vi "mqtt example gui3.vi"() -> ()   [LabVIEW 2017]
uses:
  mqtt-LabVIEW/src/class/mqtt/mqttConfigFunction.ctl
  mqtt-LabVIEW/src/class/mqtt/mqtt.lvclass/mqtt.ctl
  mqtt-LabVIEW/src/class/mqtt/mqttTypedef/mqttSubscribeCluster.ctl
  mqtt-LabVIEW/src/class/mqtt/mqttTypedef/mqttQOSlevel.ctl
  Global mqttExample.vi
  mqtt payload to double.vi
  mqtt payload to boolean.vi
  mqtt-LabVIEW/src/class/mqtt/mqtt.lvclass
panel:
  in  "G_send client time":bool
  in  "send client time":bool
  in  "auto reconnect":bool
  out "MQTT Subscribed":bool
  out "MQTT Connection":bool
  out "RX Topic":string
  out "RX Value":string
  in  "boolean control":bool
  out "boolean indicator":bool
  out "numeric indicator":dbl min=24.6 max=310.0 format="%0.3f"
  in  "send instruction":bool
  in  "numeric control":dbl format="%0.3f"
  out "messageID":u16
  out "quit":bool
  # "MQTT related"
  # "Last received message"
  # "Example program functions"
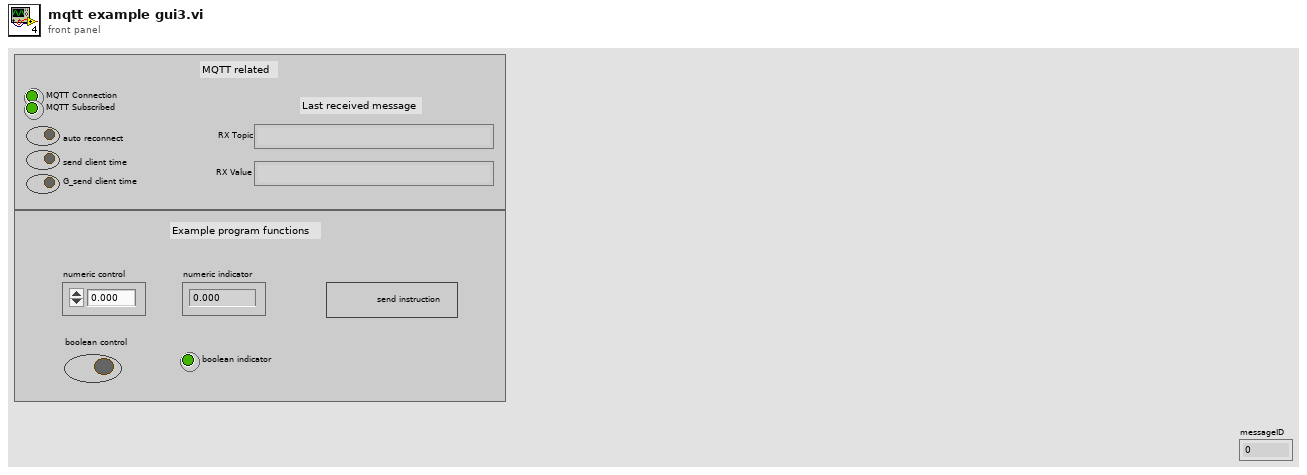
[diagram p1: front panel]
types:
  T1 = enum8{"Enabled", "Disabled", "Disabled and Grayed Out"}
  T2 = typedef "mqtt.lvclass/mqttConfigFunction.ctl" = enum16{"init", "deinit", "set", "get"}
  T3 = typedef "mqttSubscribeCluster.ctl" = cluster{"Topic":string, "QoS":T4}
  T4 = typedef "mqttQOSlevel.ctl" = enum8{"At most once", "At least once", "Exactly once", "Reserved"}
  T5 = typedef "mqttUserInformation.ctl" = cluster{"Will message":string, "Will Topic":string}
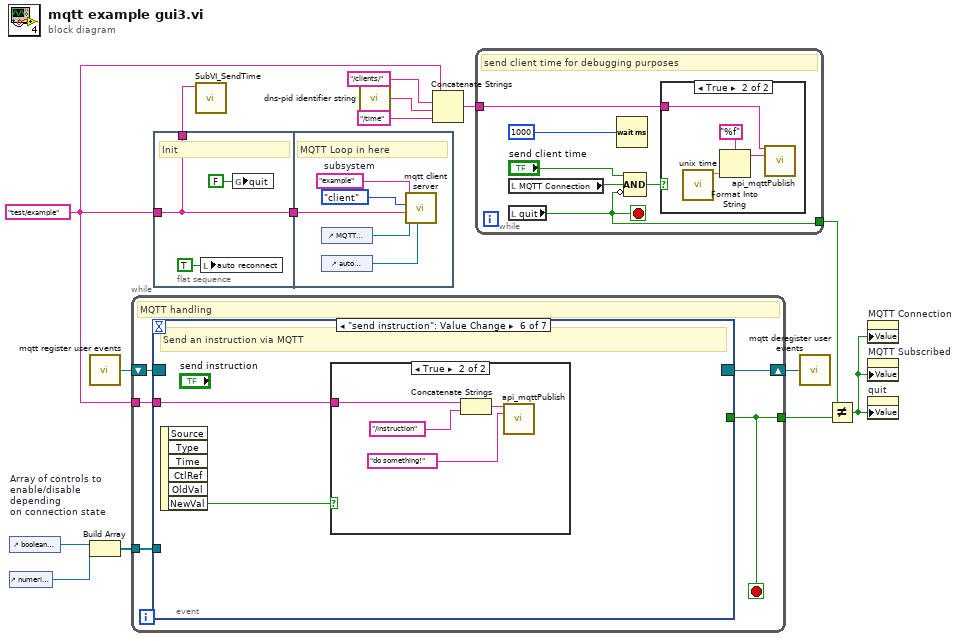
[diagram p0: block diagram]
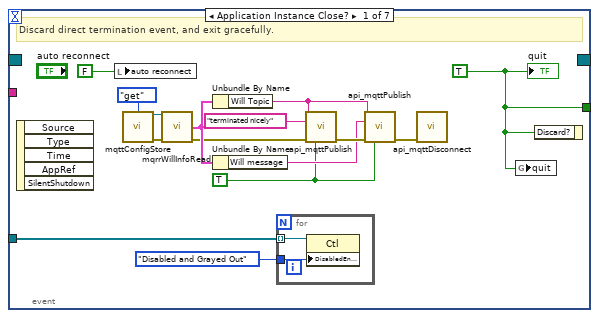
[diagram p3: hidden frame]
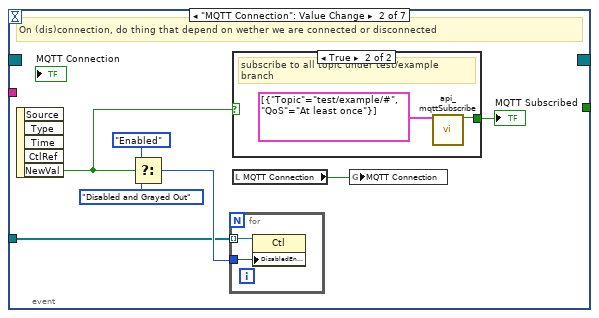
[diagram p4: hidden frame]
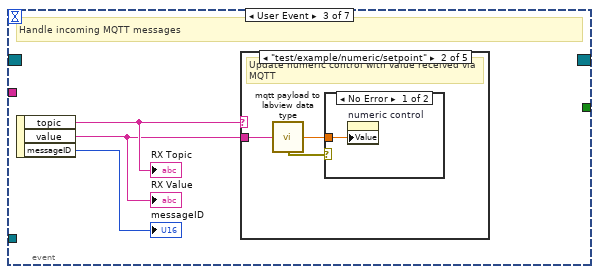
[diagram p6: hidden frame]
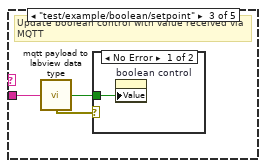
[diagram p9: hidden frame]
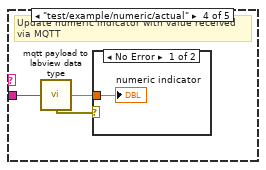
[diagram p11: hidden frame]
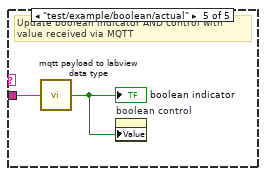
[diagram p13: hidden frame]
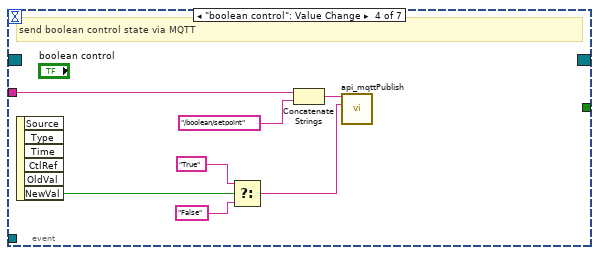
[diagram p14: hidden frame]
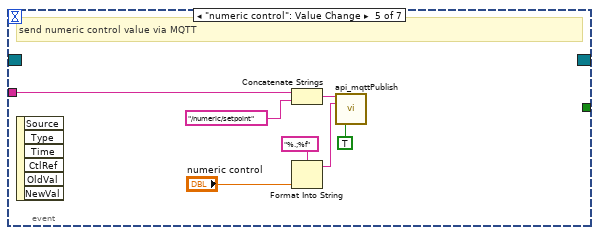
[diagram p15: hidden frame]
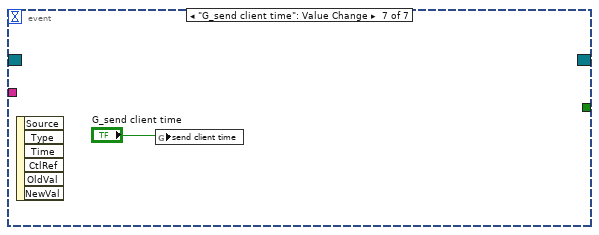
[diagram p17: hidden frame]
diagram:
  w2 = "test/example" ("mqtt prefix")
  n1 = control-ref of="boolean control"() -> (w9:refnum<vi>)
  n2 = control-ref of="numeric control"() -> (w11:refnum<vi>)
  n3 = call "mqtt register user events.vi"() -> ("Event Registration Refnum"=w15:refnum<event-registration>)  [unwired: 1 in]
  n4 = Build Array "Array of controls to \nenable/disable depending \non connection state"(w9, w11) -> (w10:refnum<vi>[])
  n5 = while {
    shift-right: [w19] -> w14
    shift-left: w15 -> [w20]
    tunnel: [w18] -> w13
    tunnel: w10 -> [w17]
    tunnel: w2 -> [w16]
    stop <- w18 stop-if-true
    # "MQTT handling"
    n6 = event shown="[5] \"send instruction\": Value Change" {
      selector: w20 -> [_ _ _ _ _ _ _]
      dyn-events: [_ _ _ _ _ _ _] -> w19
      timeout: _ -> [_ _ _ _ _ _ _]
      tunnel: [w21 _ _ _ _ _ _] -> w18
      tunnel: w16 -> [_ _ _ w67 w80 w82 _]
      tunnel: w17 -> [w28 w41 _ _ _ _ _]
      event Application Instance Close? {
        w21 = TRUE ("quit")
        w29 = TRUE ("retain(F)")
        # "Discard direct termination event, and exit gracefully."
        n7 = event-data() -> ()  [unwired: 1 in, 5 out]
        n8 = local write "auto reconnect"(FALSE ("keep connected")) -> ()
        n9 = call "mqttConfigStore.vi"("function"=mqttConfigFunction."get") -> ("mqtt.lvclass out"=w34:refnum<class "mqtt.lvclass">, "error out"=w22:errorcluster)  [unwired: 13 in]
        n10 = call "mqrrWillInfoRead.vi"("mqtt in"=w34, "error in (no error)"=w22) -> ("Will Info"=w25:T5, "error out"=w23:errorcluster)  [unwired: 11 in, 1 out]
        n11 = Unbundle By Name(w25) -> ("Will Topic"=w24:string)
        n12 = Unbundle By Name(w25) -> ("Will message"=w30:string)
        n13 = for {
          tunnel: w28 -> [w37] mode=indexing
          tunnel: T1."Disabled and Grayed Out" ("Disabled") -> [w36]
          n14 = property class="Ctl"(reference=w37, "DisabledEnum"=w36) -> ()  [unwired: 1 in, 2 out]
        }
        n15 = call "api_mqttPublish.vi"("topic"=w24, "value"="terminated nicely", "error in (no error)"=w23, "retain(F)"=w29) -> ("error out"=w32:errorcluster)  [unwired: 10 in, 1 out]
        n16 = call "api_mqttPublish.vi"("topic"=w24, "value"=w30, "error in (no error)"=w32, "retain(F)"=w29) -> ("error out"=w31:errorcluster)  [unwired: 10 in, 1 out]
        n17 = call "api_mqttDisconnect.vi"("error in (no error)"=w31) -> ()  [unwired: 13 in, 2 out]
        n18 = global write "Global mqttExample.vi" "quit"(w21) -> ()
        n19 = event-data("Discard?"=w21) -> ()  [unwired: 1 in, 1 out]
        "quit" <- w21
      }
      event "MQTT Connection": Value Change {
        # "On (dis)connection, do thing that depend on wether we are connected or disconnected"
        n20 = event-data() -> ("NewVal"=w40:bool)  [unwired: 1 in, 4 out]
        n21 = Select(t=T1."Enabled" ("Disabled"), s=w40, f=T1."Disabled and Grayed Out") -> (s? t:f=w42:T1)
        n22 = for {
          tunnel: w41 -> [w49] mode=indexing
          tunnel: w42 -> [w48]
          n23 = property class="Ctl"(reference=w49, "DisabledEnum"=w48) -> ()  [unwired: 1 in, 2 out]
        }
        n24 = case shown="True" w40 {
          selector: w40 -> [w45 _]
          tunnel: [w45 w46] -> w39
          frame False {
          }
          frame True {
            # "subscribe to all topic under test/example branch"
            n25 = call "api_mqttSubscribe.vi"("subscriptionInfo"=T3[] [{"Topic"="test/example/#", "QoS"=enum."At least once"}] ("subscriptionInfo 2")) -> ("success"=w46:bool)  [unwired: 13 in, 1 out]
          }
        }
        "MQTT Subscribed" <- w39
        n26 = local read "MQTT Connection"() -> (w38:bool)
        n27 = global write "Global mqttExample.vi" "MQTT Connection"(w38) -> ()
      }
      event User Event {
        # "Handle incoming MQTT messages"
        n28 = event-data() -> ("topic"=w51:string, "value"=w50:string, "messageID"=→"messageID":u16)  [unwired: 1 in]
        "RX Topic" <- w51
        "RX Value" <- w50
        n29 = case shown="\"test/example/numeric/setpoint\"" w51 {
          tunnel: w50 -> [_ w55 w59 w63 w66]
          frame Default {
          }
          frame "test/example/numeric/setpoint" {
            # "Update numeric control with value received via MQTT"
            n30 = call-poly "mqtt payload to labview data type.vi"("MQTT payload"=w55) -> ("double"=w54:dbl, "error out"=w53:errorcluster)  [unwired: 13 in]
            n31 = case shown="No Error" w53 {
              tunnel: w54 -> [w56 _]
              frame No Error {
                n32 = property on="numeric control" class="DigNum (strict)"("Value"=w56) -> ()  [unwired: 2 in, 2 out]
              }
              frame Error {
              }
            }
          }
          frame "test/example/boolean/setpoint" {
            # "Update boolean control with value received via MQTT"
            n33 = call-poly "mqtt payload to labview data type.vi"("String"=w59) -> ("Boolean"=w58:bool, "error out"=w57:errorcluster)  [unwired: 13 in]
            n34 = case shown="No Error" w57 {
              tunnel: w58 -> [w60 _]
              frame No Error {
                n35 = property on="boolean control" class="Bool (strict)"("Value"=w60) -> ()  [unwired: 2 in, 2 out]
              }
              frame Error {
              }
            }
          }
          frame "test/example/numeric/actual" {
            # "Update numeric indicator with value received via MQTT"
            n36 = call-poly "mqtt payload to labview data type.vi"("MQTT payload"=w63) -> ("double"=w62:dbl, "error out"=w61:errorcluster)  [unwired: 13 in]
            n37 = case shown="No Error" w61 {
              tunnel: w62 -> [w64 _]
              frame No Error {
                "numeric indicator" <- w64
              }
              frame Error {
              }
            }
          }
          frame "test/example/boolean/actual" {
            # "Update boolean indicator AND control with value received via MQTT"
            n38 = call-poly "mqtt payload to labview data type.vi"("String"=w66) -> ("Boolean"=w65:bool)  [unwired: 13 in, 1 out]
            "boolean indicator" <- w65
            n39 = property on="boolean control" class="Bool (strict)"("Value"=w65) -> ()  [unwired: 2 in, 2 out]
          }
        }
      }
      event "boolean control": Value Change {
        # "send boolean control state via MQTT"
        n40 = event-data() -> ("NewVal"=w71:bool)  [unwired: 1 in, 5 out]
        n41 = Select(t="True" ("string"), s=w71, f="False" ("string")) -> (s? t:f=w68:string)
        n42 = Concatenate Strings(w67, "/boolean/setpoint" ("string")) -> (w73:string)
        n43 = call "api_mqttPublish.vi"("topic"=w73, "value"=w68) -> ()  [unwired: 12 in, 2 out]
      }
      event "numeric control": Value Change {
        # "send numeric control value via MQTT"
        n44 = event-data() -> ()  [unwired: 1 in, 6 out]
        n45 = Concatenate Strings(w80, "/numeric/setpoint" ("string")) -> (w79:string)
        n46 = Format Into String(format string="%.;%f", "numeric control") -> (resulting string=w77:string)  [unwired: 2 in, 1 out]
        n47 = call "api_mqttPublish.vi"("topic"=w79, "value"=w77, "retain(F)"=TRUE) -> ()  [unwired: 11 in, 2 out]
      }
      event "send instruction": Value Change {
        # "Send an instruction via MQTT"
        n48 = event-data() -> ("NewVal"=w81:bool)  [unwired: 1 in, 5 out]
        n49 = case shown="True" w81 {
          tunnel: w82 -> [_ w86]
          frame False {
          }
          frame True {
            n50 = Concatenate Strings(w86, "/instruction" ("string")) -> (w85:string)
            n51 = call "api_mqttPublish.vi"("topic"=w85, "value"="do something!" ("string")) -> ()  [unwired: 12 in, 2 out]
          }
        }
      }
      event "G_send client time": Value Change {
        n52 = event-data() -> ()  [unwired: 1 in, 6 out]
        n53 = global write "Global mqttExample.vi" "send client time"("G_send client time") -> ()
      }
    }
  }
  n54 = flat-sequence {
    tunnel: [w89] -> w8
    tunnel: w2 -> [w89]
    tunnel: [w89] -> w1
    tunnel: w8 -> [w95]
    frame #0 {
      # "Init"
      n55 = local write "auto reconnect"(TRUE ("keep connected")) -> ()
      n56 = global write "Global mqttExample.vi" "quit"(FALSE ("quit")) -> ()
    }
    frame #1 {
      w93 = "example"  # subsystem
      # "MQTT Loop in here"
      n57 = control-ref of="MQTT Connection"() -> (w92:refnum<vi>)
      n58 = control-ref of="auto reconnect"() -> (w91:refnum<vi>)
      n59 = call "mqtt client server.vi"("keep connected"=w91, "connect success reference"=w92, "mqtt prefix"=w95, "client or server"=enum16{"client", "server"}."client", "subsystem"=w93) -> ()  [unwired: 6 in, 1 out]
    }
  }
  n60 = call "SubVI_SendTime.vi"("mqtt prefix"=w1) -> ()  [unwired: 11 in]
  n61 = call "dns-pid identifier string.vi"() -> ("DNS_PID Identifier string"=w5:string)  [unwired: 1 in]
  n62 = Concatenate Strings(w2, "/clients/" ("string"), w5, "/time" ("string")) -> (w7:string)
  n63 = while {
    tunnel: w7 -> [w99]
    tunnel: [w98] -> w3
    stop <- w98 stop-if-true
    # "send client time for debugging purposes"
    n64 = local read "MQTT Connection"() -> (w97:bool)
    n65 = local read "quit"() -> (w98:bool)
    n66 = Wait (ms)(milliseconds to wait=u32 1000) -> ()  [unwired: 1 out]
    n67 = Compound Arithmetic op=AND("send client time", w97, invert w98) -> (w100:bool)
    n68 = case shown="True" w100 {
      tunnel: w99 -> [_ w102]
      frame False {
      }
      frame True {
        n69 = call "unix time.vi"() -> ("Unix time"=w104:dbl)  [unwired: 10 in, 1 out]
        n70 = Format Into String(format string="%f", w104) -> (resulting string=w103:string)  [unwired: 2 in, 1 out]
        n71 = call "api_mqttPublish.vi"("topic"=w102, "value"=w103) -> ()  [unwired: 12 in, 2 out]
      }
    }
  }
  n72 = call "mqtt deregister user events.vi"("Event Registration Refnum in"=w14) -> ()  [unwired: 1 in]
  n73 = Not Equal?(x=w3, y=w13) -> (x != y?=w12:bool)
  n74 = property on="MQTT Connection" class="Bool (strict)"("Value"=w12) -> ()  [unwired: 2 in, 2 out]
  n75 = property on="MQTT Subscribed" class="Bool (strict)"("Value"=w12) -> ()  [unwired: 2 in, 2 out]
  n76 = property on="quit" class="Bool (strict)"("Value"=w12) -> ()  [unwired: 2 in, 2 out]
